vi "MeasureChannelandSend.vi"(7 "DAQChannel":refnum<k21>, 8 "error in (no error)":errorcluster, 9 "GUIMsg":T3, 10 "MainMsg":T2, 11 "QueueCluster":T1) -> (0 "error out":errorcluster)   [LabVIEW 2017]
uses:
  CTRLS/GUIMsg.ctl
  MainMsg.ctl
  CTRLS/EventCluster.ctl
  CTRLS/ListenMsg.ctl
  CTRLS/MainCluster.ctl
  CTRLS/DAQCluster.ctl
  DaqMsg.ctl
  CTRLS/GUICluster.ctl
  <vilib>/DAQmx/read.llb/DAQmx Read (Analog DBL 1Chan 1Samp).vi
  <vilib>/DAQmx/miscellaneous.llb/DAQmx Fill In Error Info.vi
  <vilib>/express/express arith-compare/Formula/XNode/ExpressFormulaBlockNode.xnode
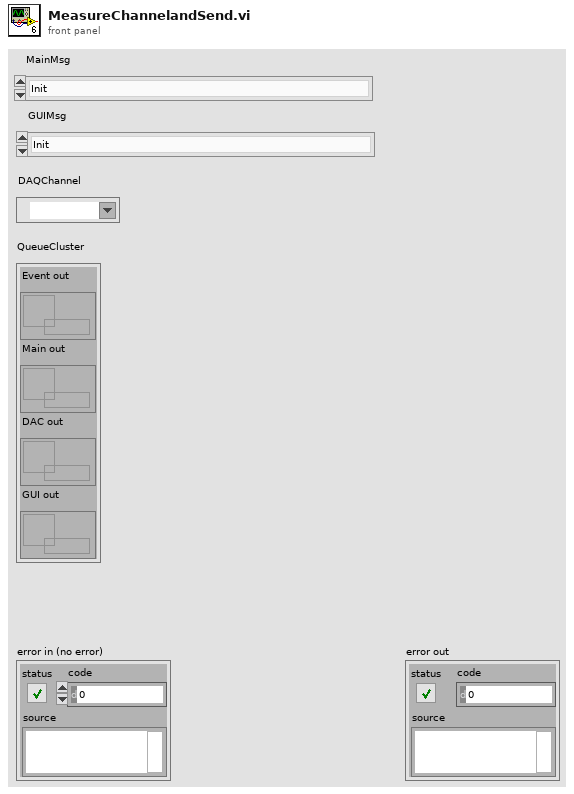
[diagram p1: front panel]
types:
  T1 = cluster{"Event out":refnum<queue>, "Main out":refnum<queue>, "DAC out":refnum<queue>, "GUI out":refnum<queue>}
  T2 = typedef "MainMsg.ctl" = enum16{"Init", "Halt", "MonitorState", "SaveState", "Filename", "AirFlow", "WaterFlow", "AirPress", "WaterPress", "WaterTemp", "NozzleForce", "SaveAll", "Error", "Supervisor"}
  T3 = typedef "GUIMsg.ctl" = enum16{"Init", "Halt", "WaterFlow", "AirFlow", "WaterPress", "AirPress", "WaterTemp", "NozzleForce", "SaveState", "MonState"}
  T4 = typedef "GUICluster.ctl" = cluster{"GUIMsg":T3, "GUINum":dbl, "GUIStr":string}
  T5 = typedef "MainCluster.ctl" = cluster{"MainMsg":T2, "MainNum":dbl, "MainStr":string}
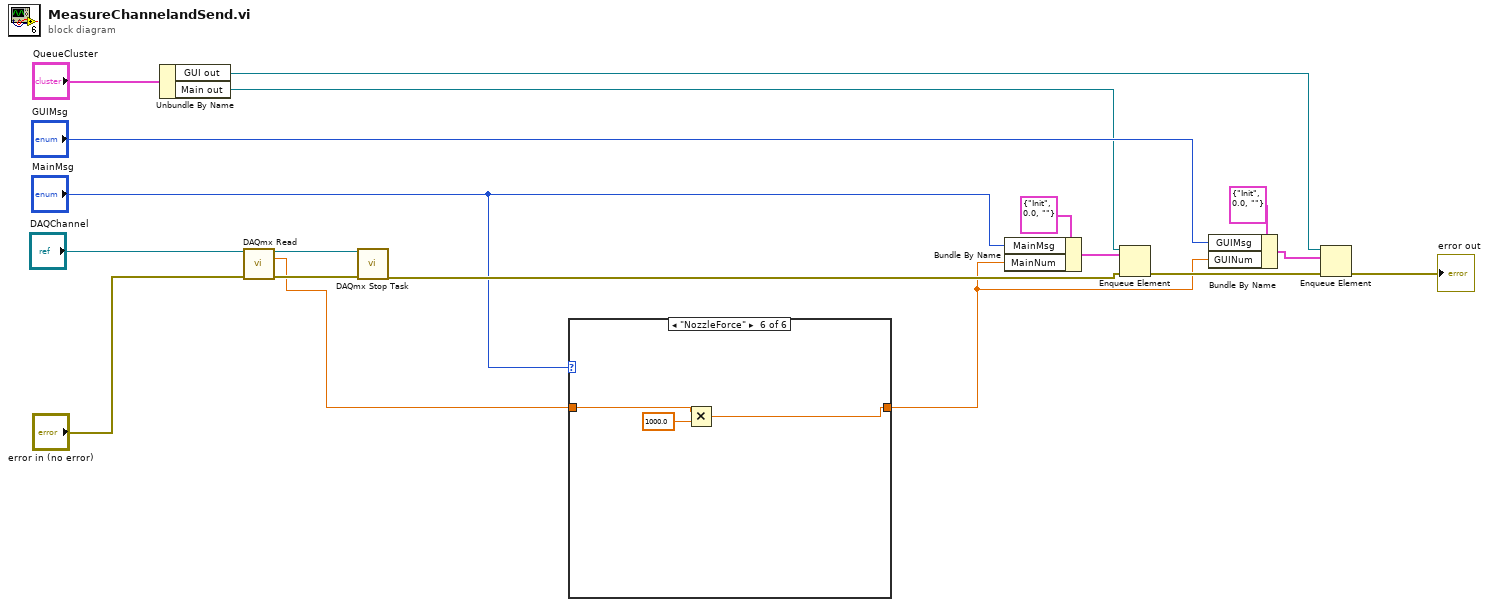
[diagram p0: block diagram]
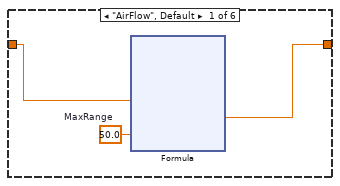
[diagram p2: hidden frame]
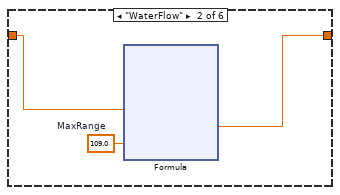
[diagram p3: hidden frame]
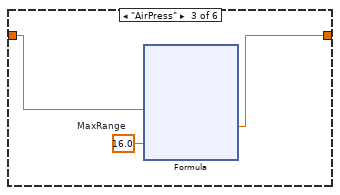
[diagram p4: hidden frame]
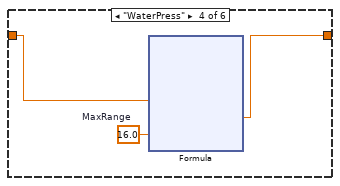
[diagram p5: hidden frame]
diagram:
  n1 = Unbundle By Name("QueueCluster") -> ("GUI out"=w14:refnum<queue>, "Main out"=w8:refnum<queue>)
  n2 = call-poly <vilib>:"DAQmx Read.vi"("task/channels in"="DAQChannel", "error in"="error in (no error)") -> ("task out"=w6:refnum<k21>, "data"=w2:dbl, "error out"=w5:errorcluster)  [unwired: 11 in]
  n3 = call <vilib>:"DAQmx Stop Task.vi"("task/channels in"=w6, "error in"=w5) -> ("error out"=w4:errorcluster)  [unwired: 12 in, 1 out]
  n4 = case shown="\"NozzleForce\"" "MainMsg" {
    tunnel: w2 -> [w21 w33 w46 w59 w71 w74]
    tunnel: [w20 w32 w45 w58 w71 w72] -> w1
    frame "AirFlow", Default {
      w19 = 50.0  # MaxRange
      n5 = xnode "Formula"("V"=w21, "Range"=w19) -> ("Result"=w20:dbl)  [unwired: 1 in, 1 out]
    }
    frame "WaterFlow" {
      w34 = 109.0  # MaxRange
      n6 = xnode "Formula"("V"=w33, "Range"=w34) -> ("Result"=w32:dbl)  [unwired: 1 in, 1 out]
    }
    frame "AirPress" {
      w47 = 16.0  # MaxRange
      n7 = xnode "Formula"("V"=w46, "Range"=w47) -> ("Result"=w45:dbl)  [unwired: 1 in, 1 out]
    }
    frame "WaterPress" {
      w60 = 16.0  # MaxRange
      n8 = xnode "Formula"("V"=w59, "Range"=w60) -> ("Result"=w58:dbl)  [unwired: 1 in, 1 out]
    }
    frame "WaterTemp" {
    }
    frame "NozzleForce" {
      n9 = Multiply(x=w74, y=1000.0) -> (x*y=w72:dbl)
    }
  }
  n10 = Bundle By Name(cluster=T5 {"MainMsg"=enum."Init", "MainNum"=0.0, "MainStr"=""} ("element"), "MainMsg"="MainMsg", "MainNum"=w1) -> (w12:T5)
  n11 = Enqueue Element(queue=w8, element=w12, error in (no error)=w4) -> (error out=w13:errorcluster)  [unwired: 1 in, 2 out]
  n12 = Bundle By Name(cluster=T4 {"GUIMsg"=enum."Init", "GUINum"=0.0, "GUIStr"=""} ("element"), "GUIMsg"="GUIMsg", "GUINum"=w1) -> (w16:T4)
  n13 = Enqueue Element(queue=w14, element=w16, error in (no error)=w13) -> (error out=→"error out":errorcluster)  [unwired: 1 in, 2 out]
